vi "UART_ConfigureSource&Capture.vi"(6 "Source Buffer":i32=1250, 7 "EOL Char (Hex)":u8=13 format="%x", 8 "error in (no error)":errorcluster, 9 "Pin Capture":string, 10 "Pin Source":string, 11 "IVI Refnum in":refnum<k15>) -> (0 "error out":errorcluster, 3 "IVI Refnum out":refnum<k15>)   [LabVIEW 2024, in "UART.lvlib"]
doc: "Configures souce and capture waveforms.\nFor UART communication the settings are:\n- 8 bit sample length\n- LSB fist\n- Serial transfer\n- EOL Char in Hexadecimal notation\n\nSource buffer specifies the length of the Source Waveform in order to overwrite it with different commands.\n\nThe name of the source waveform is hardcoded in the pattern and it's set to \"uart_source\", while the capture waveform is \"uart_capture\".\nA name change in the VI requires also a name change in the pattern"
uses:
  UART.lvlib
  <instrlib>/niDigital/niDigital.llb/niDigital Bit Order.ctl
  <instrlib>/niDigital/niDigital.llb/niDigital Data Mapping.ctl
  <instrlib>/niDigital/niDigital.llb/niDigital Create Source Waveform (Serial).vi
  <instrlib>/niDigital/niDigital.llb/niDigital Create Capture Waveform (Serial).vi
  <instrlib>/niDigital/niDigital.llb/niDigital Write Source Waveform (Broadcast U32).vi
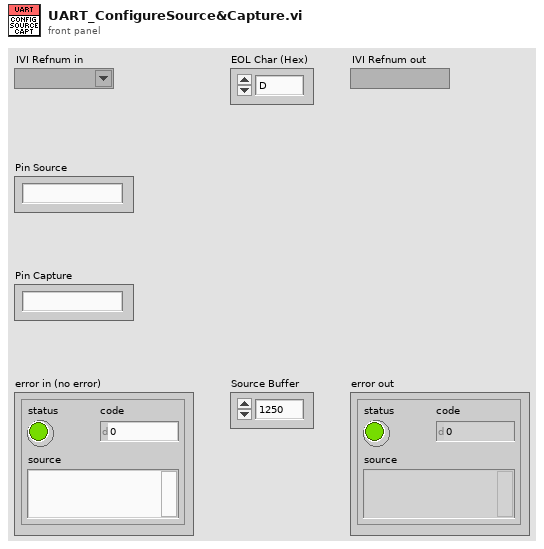
[diagram p1: front panel]
types:
  T1 = typedef "niDigital Data Mapping.ctl" = i32
  T2 = typedef "niDigital Bit Order.ctl" = i32
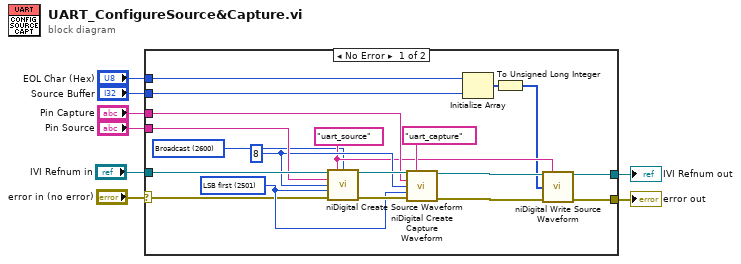
[diagram p0: block diagram]
diagram:
  n1 = case shown="No Error" "error in (no error)" {
    selector: "error in (no error)" -> [w12 w29]
    tunnel: "IVI Refnum in" -> [w25 w28]
    tunnel: "Pin Source" -> [w24 _]
    tunnel: "Pin Capture" -> [w23 _]
    tunnel: [w17 w28] -> w5
    tunnel: [w16 w29] -> w4
    tunnel: "EOL Char (Hex)" -> [w11 _]
    tunnel: "Source Buffer" -> [w10 _]
    frame No Error {
      w13 = T1 2600 items=["Broadcast"=2600, "Site Unique"=2601] ("data mapping")
      w15 = "uart_source" ("levels sheet 2")
      w21 = T2 2501 items=["MSB first"=2500, "LSB first"=2501] ("bit order")
      w22 = u32 8 ("sample width")
      n2 = call-poly <instrlib>:"niDigital Create Source Waveform.vi"("instrument handle"=w25, "waveform name"=w15, "data mapping"=w13, "pin list"=w24, "sample width"=w22, "bit order"=w21, "error in"=w12) -> ("instrument handle out"=w27:refnum<k15>, "error out"=w26:errorcluster)  [unwired: 7 in]
      n3 = call-poly <instrlib>:"niDigital Create Capture Waveform.vi"("instrument handle"=w27, "waveform name"="uart_capture" ("levels sheet"), "pin list"=w23, "sample width"=w22, "bit order"=w21, "error in"=w26) -> ("instrument handle out"=w19:refnum<k15>, "error out"=w18:errorcluster)  [unwired: 8 in]
      n4 = Initialize Array(w11, w10) -> (w14:u8[])
      n5 = To Unsigned Long Integer(number=w14) -> (unsigned 32bit integer=w9:u32[])
      n6 = call-poly <instrlib>:"niDigital Write Source Waveform.vi"("instrument handle"=w19, "waveform name"=w15, "waveform data"=w9, "error in"=w18) -> ("instrument handle out"=w17:refnum<k15>, "error out"=w16:errorcluster)  [unwired: 10 in]
    }
    frame Error {
    }
  }
  "error out" <- w4
  "IVI Refnum out" <- w5
